vi "Odour component similarity map.vi"() -> ()   [LabVIEW 2016]
panel:
  in  "odour molecule similarity map":cluster{"MDS1":dbl[], "MDS2":dbl[]}
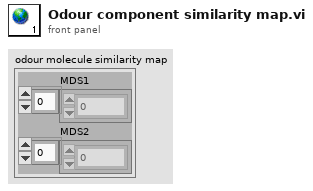
[diagram p1: front panel]
diagram:
